vi "Check if angle is in angle range - handle wrap around.vi"(9 "Angle (deg)":dbl=356.0, 10 "Angle range end (deg)":dbl=5.0, 11 "Angle range start (deg)":dbl=355.0) -> (3 "In Range?":bool=TRUE)   [LabVIEW 2013]
doc: "Checks to see if the input angle is in the angle range. Angle range goes clopckwise always so if angle start has greater magnitde than angle end, then the search goes through zero angle."
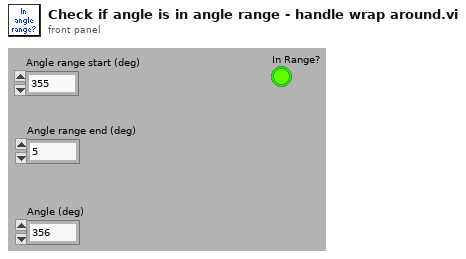
[diagram p1: front panel]
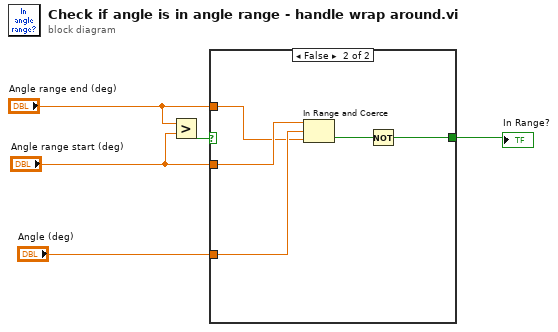
[diagram p0: block diagram]
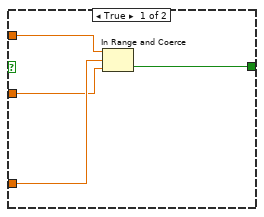
[diagram p2: hidden frame]
diagram:
  n1 = Greater?(x="Angle range end (deg)", y="Angle range start (deg)") -> (0:w5:bool)
  n2 = case shown="False" w5 {
    tunnel: "Angle range end (deg)" -> [w9 w11]
    tunnel: "Angle (deg)" -> [w8 w14]
    tunnel: "Angle range start (deg)" -> [w7 w12]
    tunnel: [w6 w10] -> w1
    frame True {
      n3 = In Range and Coerce(upper limit=w9, x=w8, lower limit=w7) -> (In Range?=w6:bool)  [unwired: 1 out]
    }
    frame False {
      n4 = In Range and Coerce(upper limit=w12, x=w14, lower limit=w11) -> (In Range?=w13:bool)  [unwired: 1 out]
      n5 = Not(x=w13) -> (.not. x?=w10:bool)
    }
  }
  "In Range?" <- w1
